vi "Encode YAML.vi"(8 "error in (no error)":errorcluster, 11 "YAML Parser in":refnum<class "YAML Parser.lvclass">) -> (0 "error out":errorcluster, 2 "YAML String":string, 3 "YAML Parser out":refnum<class "YAML Parser.lvclass">)   [LabVIEW 2015, in "YAML Parser.lvclass"]
uses:
  YAML Parser.lvclass
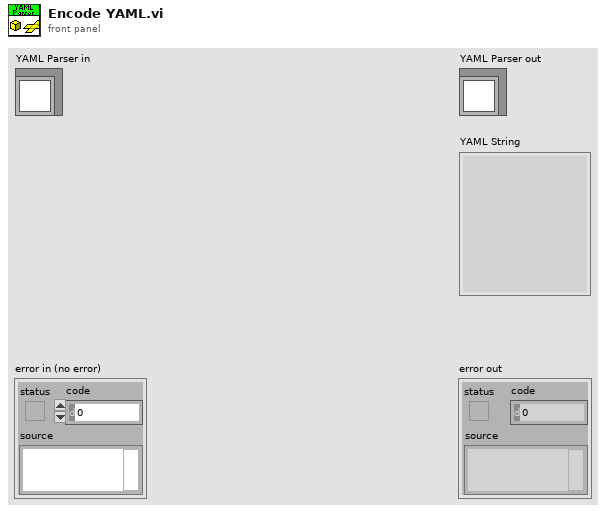
[diagram p1: front panel]
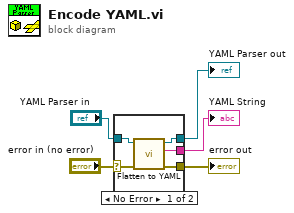
[diagram p0: block diagram]
diagram:
  n1 = case shown="No Error" "error in (no error)" {
    selector: "error in (no error)" -> [w10 w12]
    tunnel: [w9 w12] -> w4
    tunnel: [w6 w11] -> w2
    tunnel: "YAML Parser in" -> [w7 w11]
    tunnel: [w8 _] -> w1
    frame No Error {
      n2 = call "Flatten to YAML.vi"("error in (no error)"=w10, "YAML Parser in"=w7) -> ("error out"=w9:errorcluster, "YAML String"=w8:string, "YAML Parser out"=w6:refnum<class "YAML Parser.lvclass">)  [unwired: 7 in]
    }
    frame Error {
    }
  }
  "error out" <- w4
  "YAML Parser out" <- w2
  "YAML String" <- w1
